vi "2-input NOT.vi"(10 "Obtained Expression":string, 11 "Input List":string[](array[string])) -> (1 "O/p = I/p":string, 2 "NOT ?":bool, 3 "Logic Exp":string)   [LabVIEW 2014]
doc: "This VI is used to compare the obtained logic with the logic of NAND gate."
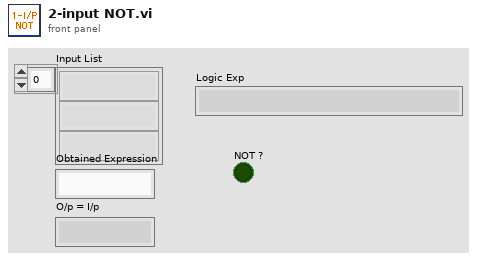
[diagram p1: front panel]
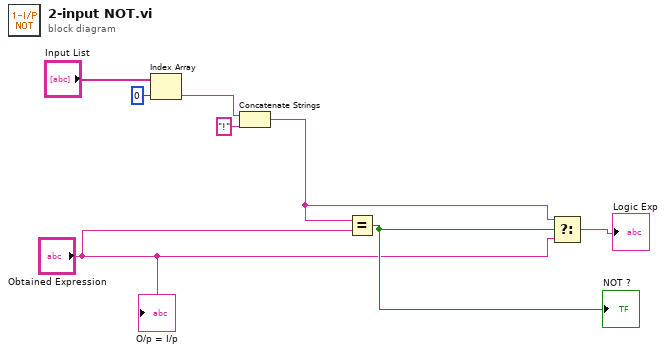
[diagram p0: block diagram]
diagram:
  n1 = Index Array(array="Input List", index=0) -> (element=w8:string)
  n2 = Concatenate Strings(w8, "!" ("t")) -> (w1:string)
  n3 = Equal?(x=w1, y="Obtained Expression") -> (x = y?=w6:bool)
  "NOT ?" <- w6
  n4 = Select(t=w1, s=w6, f="Obtained Expression") -> (s? t:f=→"Logic Exp":string)
  "O/p = I/p" <- "Obtained Expression"
